vi "Q8381 SPAN_FULL.vi"(1 "GPIB Address":u16=8 max=31 step=1, 2 "VISA resource name":refnum<visa-resource-name>) -> (0 "GPIB Status":bool)   [LabVIEW 2017]
panel:
  out "Program Code":string
  # "SPAN__FULL"
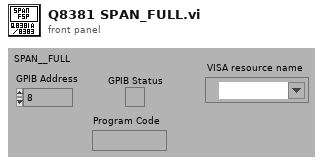
[diagram p1: front panel]
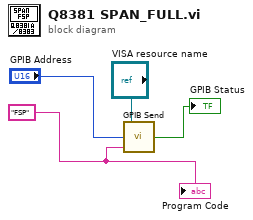
[diagram p0: block diagram]
diagram:
  w1 = "FSP"
  n1 = call "GPIB Send.vi"("Command String"=w1, "Address"="GPIB Address", "VISA resource name"="VISA resource name") -> ("Error"=→"GPIB Status":bool)
  "Program Code" <- w1
